vi "ProcessBufferUpdates.vi"(11 "MockGyroData":T1={"BufferUpdateFIFO"="MockGyroBufferUpdate", "MockGyroCommandInput"="ModbusSubnetEGyroRxDataFIFO", "MockGyroDataOutput"="ModbusSubnetEGyroTxDataFIFO", "MockGyroDataRate"="MockGyroDataRateRegister", "MockGyroXValue"="MockGyroXValueRegister", "MockGyroYValue"="MockGyroYValueRegister", "MockGyroZValue"="MockGyroZValueRegister", "MockGyroStatus"="MockGyroStatusRegister", "MockGyroTemperature"="MockGyroTemperatureRegister", "CRCDataFIFO"="MockGyroCRCDataFIFO", "CRCCalculateFIFO"="MockGyroCRCCalculateFIFO", "CRCFIFO"="MockGyroCRCFIFO", "MockGyroCommandReplyFIFO"="MockGyroCommandReplyFIFO", "MockGyroReplyReadyFIFO"="MockGyroReplyReadyFIFO", "MockGyroModeFIFO"="MockGyroModeFIFO"}) -> ()   [LabVIEW 2016, in "FPGAMockGyro.lvlib"]
uses:
  FPGAMockGyro.lvlib
  DataTypes/MockGyroData.ctl
  DataTypes/MockGyroBufferUpdateData.ctl
  DataTypes/MockGyroBufferUpdateStates.ctl
  <vilib>/Platform/TimedLoop/XDataNode/timing_clust.ctl
  <vilib>/Platform/TimedLoop/XDataNode/nitl_modes.ctl
  <vilib>/Platform/TimedLoop/XDataNode/wakeup.ctl
  <vilib>/rvi/Emulation/niFpgaSctlEmulationGetInTimedLoop.vi
  <vilib>/rvi/Emulation/niFpgaEmulationReportErrorSimple.vi
  <vilib>/rvi/Emulation/niFpgaGetClockAttributes.vi
  <vilib>/rvi/Emulation/niFpgaCriticalErrorInLSC.vi
  <vilib>/rvi/DataTransferAndStorage/Container/Common/niFpgaContainerExecOnDevCompGetState.vi
  <vilib>/rvi/Emulation/niFpgaEmulationIsFPGAContextNoSignature.vi
  <vilib>/rvi/errors/niFpgaSetErrorForExecOnDevCompSimple.vi
  <vilib>/rvi/eio/common/nirviEmuReportErrorAndStop.vi
  <vilib>/rvi/DataTransferAndStorage/Container/Common/niFpgaContainerGetUniqueNameForEmu.vi
  <vilib>/rvi/FIFO/Fifo_Resource/nirvififoEmulationSetSize.vi
  <vilib>/rvi/FIFO/Fifo_Resource/nirviFifoEmulationQueueMgr.vi
  <instcachedir>/0/nirviFifoEmulationQueueMgr_E5CAEC123FF24DC58D834DCA3CDAA9B5.lvgen/nirviFifoEmulationQueueMgr_E5CAEC123FF24DC58D834DCA3CDAA9B5_000.vi
  <vilib>/rvi/FIFO/Fifo_Resource/nirvififoEmulationDetermineInputValidOut.vi
  <vilib>/rvi/FIFO/Fifo_Resource/nirvififoEmulationCreateLock.vi
  <vilib>/rvi/Emulation/niFpgaProcessEmulError.vi
  <vilib>/rvi/FIFO/Fifo_Resource/nirvififoEmulationObtainLock.vi
  <vilib>/rvi/FIFO/Fifo_Resource/nirvififoEmulationReleaseLock.vi
  <vilib>/rvi/occurrence/nirviWaitOnOccurrenceBase.vi
  <vilib>/rvi/errors/nirviReportUnexpectedCaseInternalError.vi
  <vilib>/rvi/errors/nirviReportUnexpectedCaseInternalError (U32).vi
  <vilib>/Utility/error.llb/Clear Errors.vi
  <vilib>/rvi/interface/RandomDataEmulation/niFpgaRandomDataHandleErrors.vi
  <vilib>/rvi/Memory/Memory_Emulation/niFpgaMemoryEmulationCacheClearOnFirstRun.vi
  <vilib>/rvi/Memory/Memory_Emulation/nirvimemoryEmulationManagerCache_MakeExclusive.vi
  <vilib>/rvi/Memory/Memory_Emulation/niFpgaMemoryEmulationValidateCache.vi
  <vilib>/rvi/Memory/Memory_Emulation/nirvimemoryEmulationManagerCache_InsertValue.vi
  <vilib>/rvi/Memory/Memory_Emulation/nirvimemoryEmulationManagerCache_ReleaseExclusive.vi
  <vilib>/rvi/Memory/Memory_Emulation/nirvimemoryEmulationManagerCache_GetValue.vi
  <vilib>/rvi/Memory/Memory_Emulation/nirvimemoryEmulationManagerCache_SetValue.vi
  <vilib>/Platform/TimedLoop/XDataNode/XDataNode.xnode
  <vilib>/rvi/DataTransferAndStorage/Container/XNode/niFpgaContainer.xnode
  <vilib>/rvi/FIFO/Fifo_Resource/niFpgaFifoEmulationRefIn.vi
  <vilib>/rvi/DataTransferAndStorage/Register/Emulation/niFpgaRegisterEmulationRefIn.vi
  <vilib>/Platform/TimedLoop/XDataNode/XDNodeRunTimeDep.lvlib
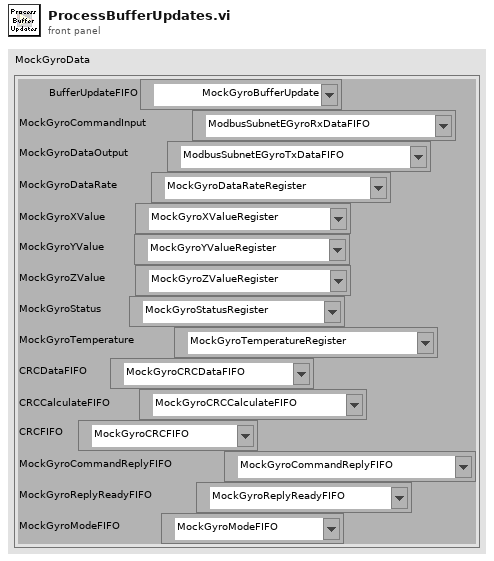
[diagram p1: front panel]
types:
  T1 = typedef "FPGAMockGyro.lvlib/MockGyroData.ctl" = cluster{"BufferUpdateFIFO":refnum<k21>, "MockGyroCommandInput":refnum<k21>, "MockGyroDataOutput":refnum<k21>, "MockGyroDataRate":refnum<k21>, "MockGyroXValue":refnum<k21>, "MockGyroYValue":refnum<k21>, "MockGyroZValue":refnum<k21>, "MockGyroStatus":refnum<k21>, "MockGyroTemperature":refnum<k21>, "CRCDataFIFO":refnum<k21>, "CRCCalculateFIFO":refnum<k21>, "CRCFIFO":refnum<k21>, "MockGyroCommandReplyFIFO":refnum<k21>, "MockGyroReplyReadyFIFO":refnum<k21>, "MockGyroModeFIFO":refnum<k21>}
  T2 = typedef "FPGAMockGyro.lvlib/MockGyroBufferUpdateData.ctl" = cluster{"BufferUpdateLoopStates":T3, "Status":u8, "XValue":u32, "YValue":u32, "ZValue":u32, "Temperature":u16, "Index":i16}
  T3 = typedef "FPGAMockGyro.lvlib/MockGyroBufferUpdateStates.ctl" = enum8{"ReadX", "ReadY", "ReadZ", "ReadStatus", "ReadTemperature", "WriteValues"}
  T4 = typedef "XDNodeRunTimeDep.lvlib/timing_clust.ctl" = cluster{"Expected End [f-1]":u64, "Actual End [f-1]":u64, "Finished Late? [f-1]":bool, "Expected End [i-1]":u64, "Actual End [i-1]":u64, "Finished Late? [i-1]":bool, "Expected Start [i]":u64, "Actual Start [i]":u64, "Expected Start [f]":u64, "Actual Start [f]":u64, "Source Name":string, "Structure Name":string, "Period":i64, "Deadline":i64, "Offset":i64, "Start":i64, "Priority":i32, "Timeout":i32, "Mode":T5, "Wakeup Reason":T6, "Error":errorcluster, "Source Type":string, "Secondary Source Type":string, "Global End Time":u64, "Global Start Time":u64, "Frame Duration":u64, "Iteration Duration":u64, "Assigned CPU":i32, "I/O Scan Engine Mode":u32}
  T5 = typedef "XDNodeRunTimeDep.lvlib/nitl_modes.ctl" = enum32{"No Change", "Process missed periods, maintain original phase", "Discard missed periods, maintain original phase", "Process missed periods, ignore original phase", "Discard missed periods, ignore original phase"}
  T6 = typedef "XDNodeRunTimeDep.lvlib/wakeup.ctl" = enum32{"Normal", "Aborted", "Asynchronous wakeup", "Timing source error", "Timed loop error", "Timeout"}
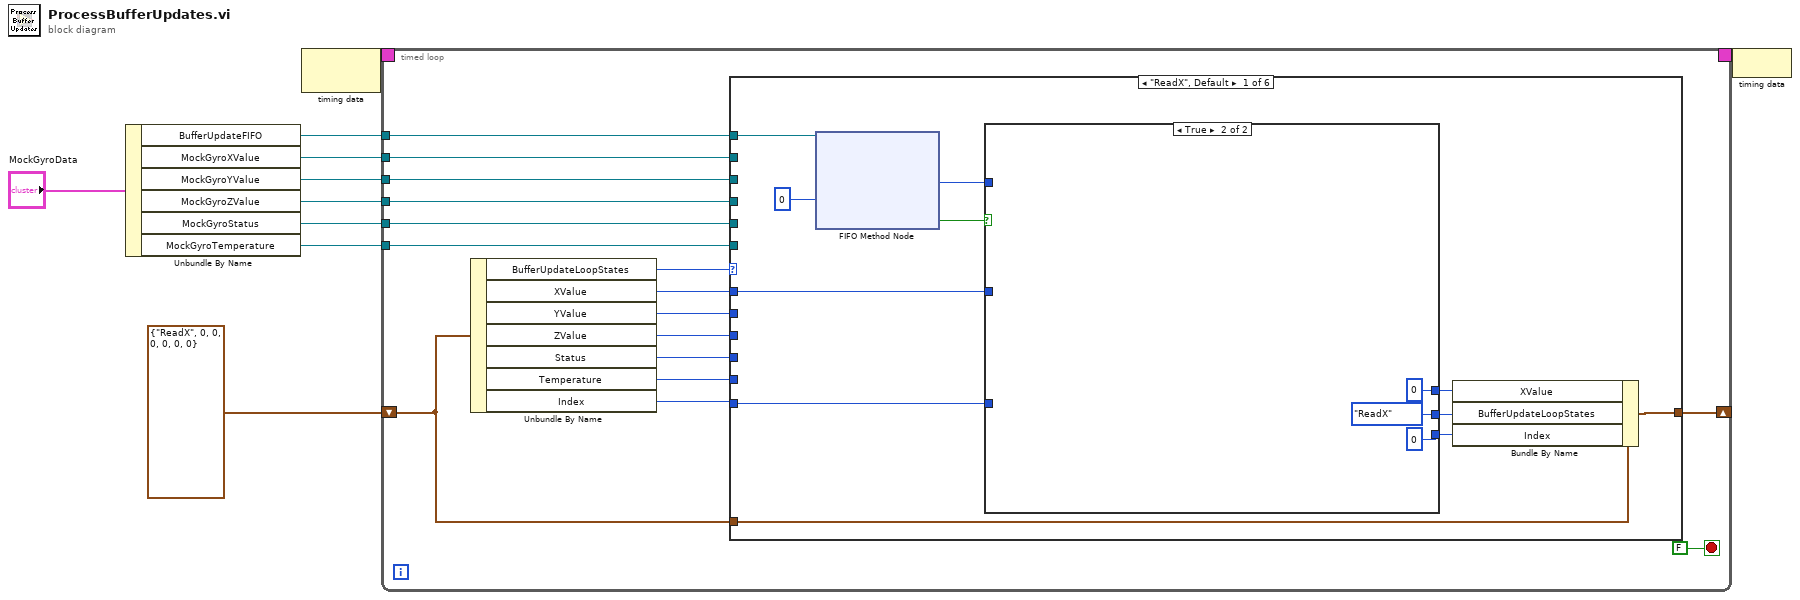
[diagram p0: block diagram]
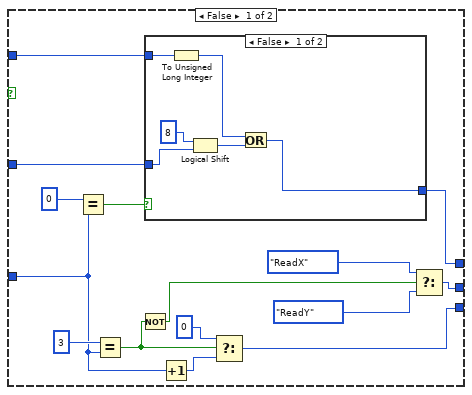
[diagram p2: hidden frame]
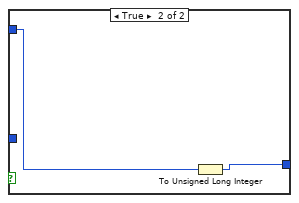
[diagram p3: hidden frame]
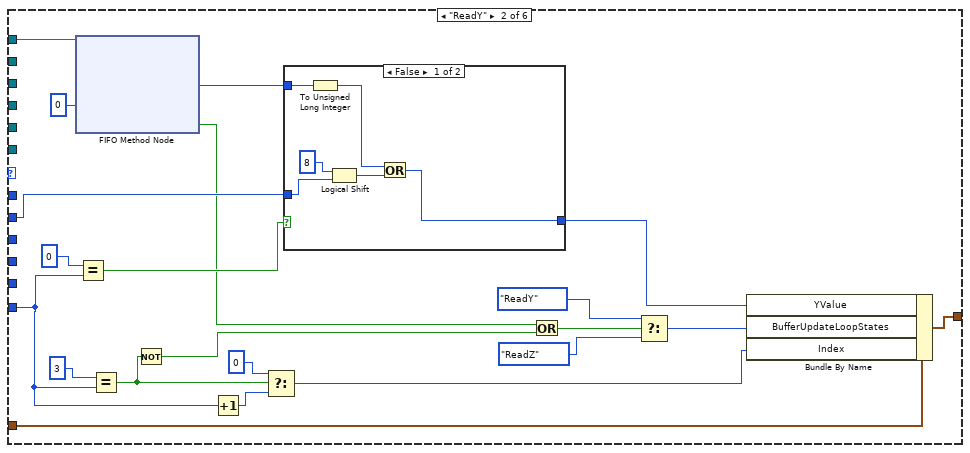
[diagram p4: hidden frame]
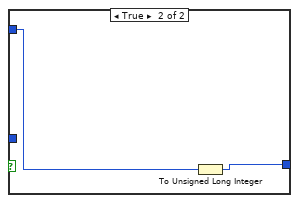
[diagram p5: hidden frame]
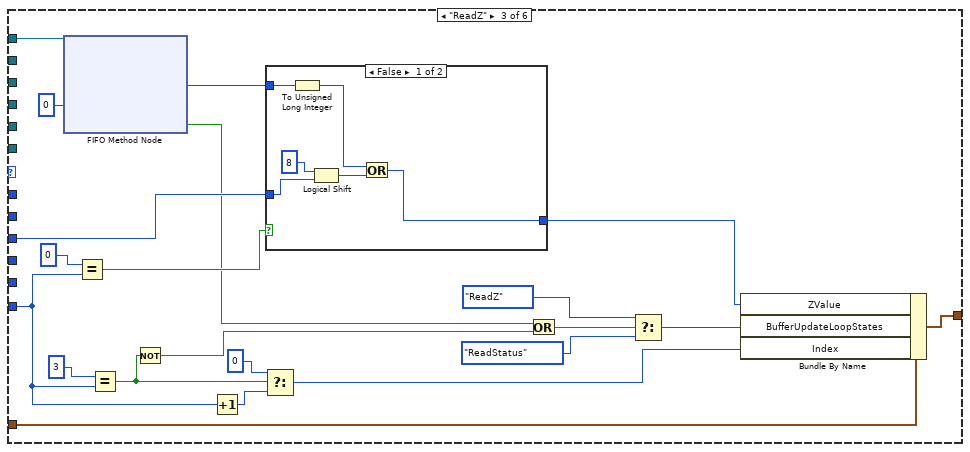
[diagram p6: hidden frame]
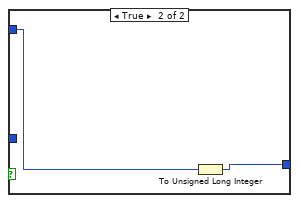
[diagram p7: hidden frame]
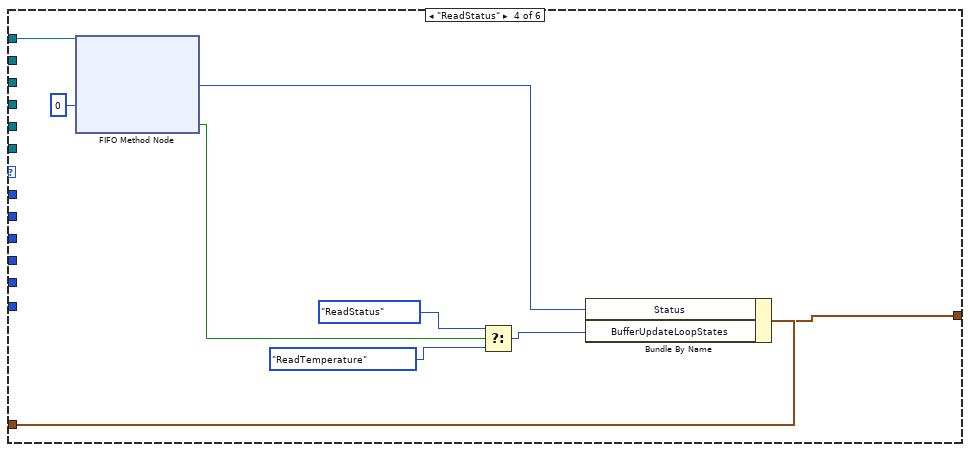
[diagram p8: hidden frame]
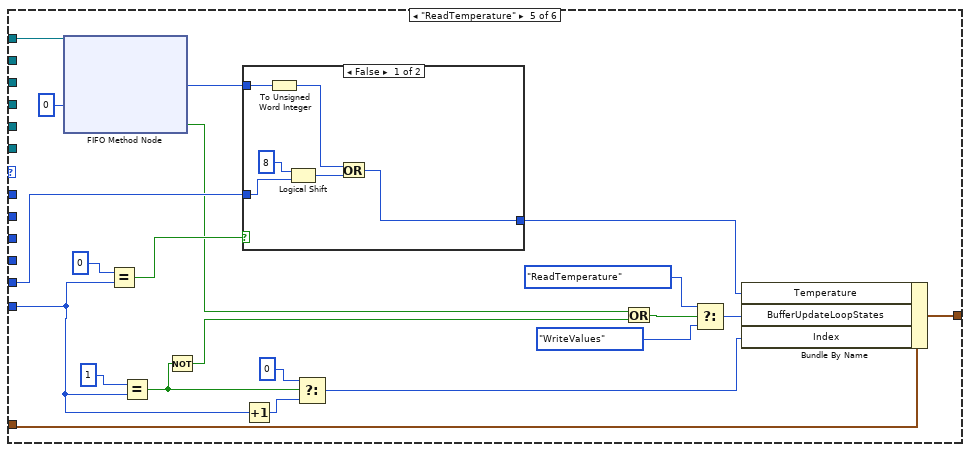
[diagram p9: hidden frame]
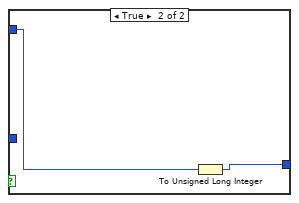
[diagram p10: hidden frame]
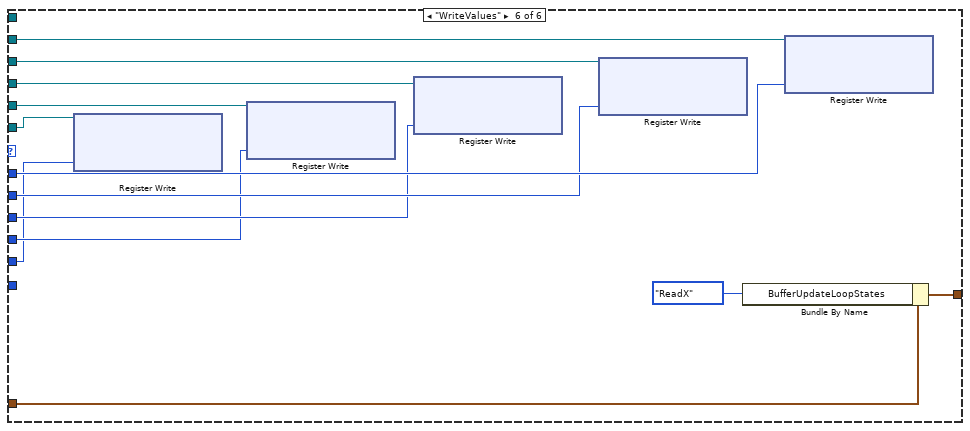
[diagram p11: hidden frame]
diagram:
  n1 = Unbundle By Name("MockGyroData") -> ("BufferUpdateFIFO"=w6:refnum<k21>, "MockGyroXValue"=w5:refnum<k21>, "MockGyroYValue"=w4:refnum<k21>, "MockGyroZValue"=w3:refnum<k21>, "MockGyroStatus"=w2:refnum<k21>, "MockGyroTemperature"=w1:refnum<k21>)
  n2 = node-c288() -> (w9:T4)  [unwired: 1 in]
  n3 = timed-loop {
    timing: w9 -> [_]
    timing-out: [_] -> w8
    shift-right: [w23] -> _
    shift-left: T2 {"BufferUpdateLoopStates"=enum."ReadX", "Status"=0, "XValue"=0, "YValue"=0, "ZValue"=0, "Temperature"=0, "Index"=0} ("BufferUpdateLoopData") -> [w24]
    tunnel: w6 -> [w25]
    tunnel: w5 -> [w22]
    tunnel: w4 -> [w21]
    tunnel: w3 -> [w20]
    tunnel: w2 -> [w19]
    tunnel: w1 -> [w18]
    stop <- FALSE stop-if-true
    n4 = Unbundle By Name(w24) -> ("BufferUpdateLoopStates"=w17:T3, "XValue"=w15:u32, "YValue"=w14:u32, "ZValue"=w13:u32, "Status"=w12:u8, "Temperature"=w11:u16, "Index"=w16:i16)
    n5 = case shown="\"ReadX\", Default" w17 {
      tunnel: w25 -> [w37 w84 w110 w130 w151 _]
      tunnel: w24 -> [w35 w83 w109 w127 w150 w170]
      tunnel: [w33 w82 w108 w126 w149 w172] -> w23
      tunnel: w22 -> [_ _ _ _ _ w169]
      tunnel: w21 -> [_ _ _ _ _ w167]
      tunnel: w20 -> [_ _ _ _ _ w165]
      tunnel: w19 -> [_ _ _ _ _ w163]
      tunnel: w18 -> [_ _ _ _ _ w161]
      tunnel: w16 -> [w30 w73 w101 _ w137 _]
      tunnel: w15 -> [w28 _ _ _ _ w168]
      tunnel: w14 -> [_ w71 _ _ _ w166]
      tunnel: w13 -> [_ _ w99 _ _ w164]
      tunnel: w12 -> [_ _ _ _ _ w162]
      tunnel: w11 -> [_ _ _ _ w136 w160]
      frame "ReadX", Default {
        n6 = xnode ("FIFO Method Node")("Timeout"=0, "FIFO In"=w37) -> ("Element"=w32:u8, "Timed Out?"=w27:bool)  [unwired: 1 out]
        n7 = case shown="True" w27 {
          tunnel: [w50 MockGyroBufferUpdateStates."ReadX" ("BufferUpdateLoopStates")] -> w34
          tunnel: w32 -> [w47 _]
          tunnel: [w46 u32 0] -> w31
          tunnel: w30 -> [w42 _]
          tunnel: [w41 i16 0 ("t")] -> w29
          tunnel: w28 -> [w38 _]
          frame False {
            n8 = Equal?(x=i16 0, y=w42) -> (x = y?=w48:bool)
            n9 = Equal?(x=i16 3 ("y"), y=w42) -> (x = y?=w40:bool)
            n10 = Not(x=w40) -> (.not. x?=w39:bool)
            n11 = case shown="False" w48 {
              tunnel: w47 -> [w55 w60]
              tunnel: [w53 w59] -> w46
              tunnel: w38 -> [w58 _]
              frame False {
                n12 = To Unsigned Long Integer(number=w55) -> (unsigned 32bit integer=w54:u32)
                n13 = Logical Shift(y=i16 8, x=w58) -> (x << y=w56:u32)
                n14 = Or(x=w54, y=w56) -> (x .or. y?=w53:u32)
              }
              frame True {
                n15 = To Unsigned Long Integer(number=w60) -> (unsigned 32bit integer=w59:u32)
              }
            }
            n16 = Increment(x=w42) -> (x+1=w43:i16)
            n17 = Select(t=i16 0, s=w40, f=w43) -> (s? t:f=w41:i16)
            n18 = Select(t=MockGyroBufferUpdateStates."ReadX" ("BufferUpdateLoopStates"), s=w39, f=MockGyroBufferUpdateStates."ReadY" ("BufferUpdateLoopStates")) -> (s? t:f=w50:T3)
          }
          frame True {
          }
        }
        n19 = Bundle By Name(cluster=w35, "XValue"=w31, "BufferUpdateLoopStates"=w34, "Index"=w29) -> (w33:T2)
      }
      frame "ReadY" {
        n20 = xnode ("FIFO Method Node")("Timeout"=0, "FIFO In"=w84) -> ("Element"=w72:u8, "Timed Out?"=w68:bool)  [unwired: 1 out]
        n21 = Equal?(x=i16 0, y=w73) -> (x = y?=w70:bool)
        n22 = Equal?(x=i16 3 ("y"), y=w73) -> (x = y?=w74:bool)
        n23 = Not(x=w74) -> (.not. x?=w69:bool)
        n24 = Increment(x=w73) -> (x+1=w65:i16)
        n25 = Select(t=i16 0, s=w74, f=w65) -> (s? t:f=w64:i16)
        n26 = case shown="False" w70 {
          tunnel: w72 -> [w87 w92]
          tunnel: [w85 w91] -> w66
          tunnel: w71 -> [w90 _]
          frame False {
            n27 = To Unsigned Long Integer(number=w87) -> (unsigned 32bit integer=w86:u32)
            n28 = Logical Shift(y=i16 8, x=w90) -> (x << y=w88:u32)
            n29 = Or(x=w86, y=w88) -> (x .or. y?=w85:u32)
          }
          frame True {
            n30 = To Unsigned Long Integer(number=w92) -> (unsigned 32bit integer=w91:u32)
          }
        }
        n31 = Or(x=w68, y=w69) -> (x .or. y?=w67:bool)
        n32 = Select(t=MockGyroBufferUpdateStates."ReadY", s=w67, f=MockGyroBufferUpdateStates."ReadZ" ("BufferUpdateLoopStates")) -> (s? t:f=w80:T3)
        n33 = Bundle By Name(cluster=w83, "YValue"=w66, "BufferUpdateLoopStates"=w80, "Index"=w64) -> (w82:T2)
      }
      frame "ReadZ" {
        n34 = xnode ("FIFO Method Node")("Timeout"=0, "FIFO In"=w110) -> ("Element"=w98:u8, "Timed Out?"=w96:bool)  [unwired: 1 out]
        n35 = Equal?(x=i16 0, y=w101) -> (x = y?=w100:bool)
        n36 = Equal?(x=i16 3 ("y"), y=w101) -> (x = y?=w102:bool)
        n37 = Not(x=w102) -> (.not. x?=w97:bool)
        n38 = Increment(x=w101) -> (x+1=w103:i16)
        n39 = Select(t=i16 0, s=w102, f=w103) -> (s? t:f=w94:i16)
        n40 = case shown="False" w100 {
          tunnel: w98 -> [w116 w121]
          tunnel: [w114 w120] -> w93
          tunnel: w99 -> [w119 _]
          frame False {
            n41 = To Unsigned Long Integer(number=w116) -> (unsigned 32bit integer=w115:u32)
            n42 = Logical Shift(y=i16 8, x=w119) -> (x << y=w117:u32)
            n43 = Or(x=w115, y=w117) -> (x .or. y?=w114:u32)
          }
          frame True {
            n44 = To Unsigned Long Integer(number=w121) -> (unsigned 32bit integer=w120:u32)
          }
        }
        n45 = Or(x=w96, y=w97) -> (x .or. y?=w95:bool)
        n46 = Select(t=MockGyroBufferUpdateStates."ReadZ", s=w95, f=MockGyroBufferUpdateStates."ReadStatus" ("BufferUpdateLoopStates")) -> (s? t:f=w112:T3)
        n47 = Bundle By Name(cluster=w109, "ZValue"=w93, "BufferUpdateLoopStates"=w112, "Index"=w94) -> (w108:T2)
      }
      frame "ReadStatus" {
        n48 = xnode ("FIFO Method Node")("Timeout"=0, "FIFO In"=w130) -> ("Element"=w128:u8, "Timed Out?"=w123:bool)  [unwired: 1 out]
        n49 = Select(t=MockGyroBufferUpdateStates."ReadStatus", s=w123, f=MockGyroBufferUpdateStates."ReadTemperature" ("t")) -> (s? t:f=w124:T3)
        n50 = Bundle By Name(cluster=w127, "Status"=w128, "BufferUpdateLoopStates"=w124) -> (w126:T2)
      }
      frame "ReadTemperature" {
        n51 = xnode ("FIFO Method Node")("Timeout"=0, "FIFO In"=w151) -> ("Element"=w144:u8, "Timed Out?"=w133:bool)  [unwired: 1 out]
        n52 = Equal?(x=i16 0, y=w137) -> (x = y?=w135:bool)
        n53 = Equal?(x=i16 1 ("y"), y=w137) -> (x = y?=w138:bool)
        n54 = Not(x=w138) -> (.not. x?=w134:bool)
        n55 = case shown="False" w135 {
          tunnel: w144 -> [w154 w159]
          tunnel: [w152 w158] -> w143
          tunnel: w136 -> [w157 _]
          frame False {
            n56 = To Unsigned Word Integer(number=w154) -> (unsigned 16bit integer=w153:u16)
            n57 = Logical Shift(y=i16 8, x=w157) -> (x << y=w155:u16)
            n58 = Or(x=w153, y=w155) -> (x .or. y?=w152:u16)
          }
          frame True {
            n59 = To Unsigned Long Integer(number=w159) -> (unsigned 32bit integer=w158:u32)
          }
        }
        n60 = Increment(x=w137) -> (x+1=w139:i16)
        n61 = Select(t=i16 0, s=w138, f=w139) -> (s? t:f=w131:i16)
        n62 = Or(x=w133, y=w134) -> (x .or. y?=w132:bool)
        n63 = Select(t=MockGyroBufferUpdateStates."ReadTemperature", s=w132, f=MockGyroBufferUpdateStates."WriteValues" ("t")) -> (s? t:f=w147:T3)
        n64 = Bundle By Name(cluster=w150, "Temperature"=w143, "BufferUpdateLoopStates"=w147, "Index"=w131) -> (w149:T2)
      }
      frame "WriteValues" {
        n65 = xnode ("Register Write")("Data"=w160, "Register In"=w161) -> ()  [unwired: 1 out]
        n66 = xnode ("Register Write")("Data"=w162, "Register In"=w163) -> ()  [unwired: 1 out]
        n67 = xnode ("Register Write")("Data"=w164, "Register In"=w165) -> ()  [unwired: 1 out]
        n68 = xnode ("Register Write")("Data"=w166, "Register In"=w167) -> ()  [unwired: 1 out]
        n69 = Bundle By Name(cluster=w170, "BufferUpdateLoopStates"=MockGyroBufferUpdateStates."ReadX") -> (w172:T2)
        n70 = xnode ("Register Write")("Data"=w168, "Register In"=w169) -> ()  [unwired: 1 out]
      }
    }
  }
  n71 = node-c288(w8) -> ()
